vi "Array_size.vi"() -> ()   [LabVIEW 2013]
panel:
  out "Array size":u32[](array[numeric])
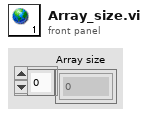
[diagram p1: front panel]
diagram:
